vi "OpenFile_windows.vi"(0 "文件完整路径":path, 3 "文件父路径":path, 5 "文件全称":string) -> ()   [LabVIEW 2019]
panel:
  # "优先识别完整路径\n完整路径错误再识别拼接路径"
  # "用CMD来打开指定的文件，只要电脑的默认打开方式能打开对应的文件"
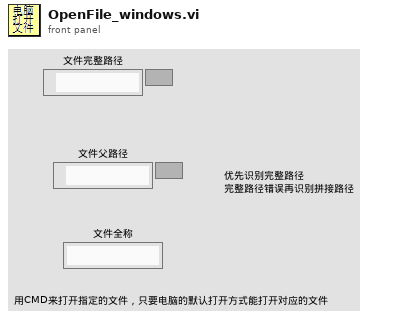
[diagram p1: front panel]
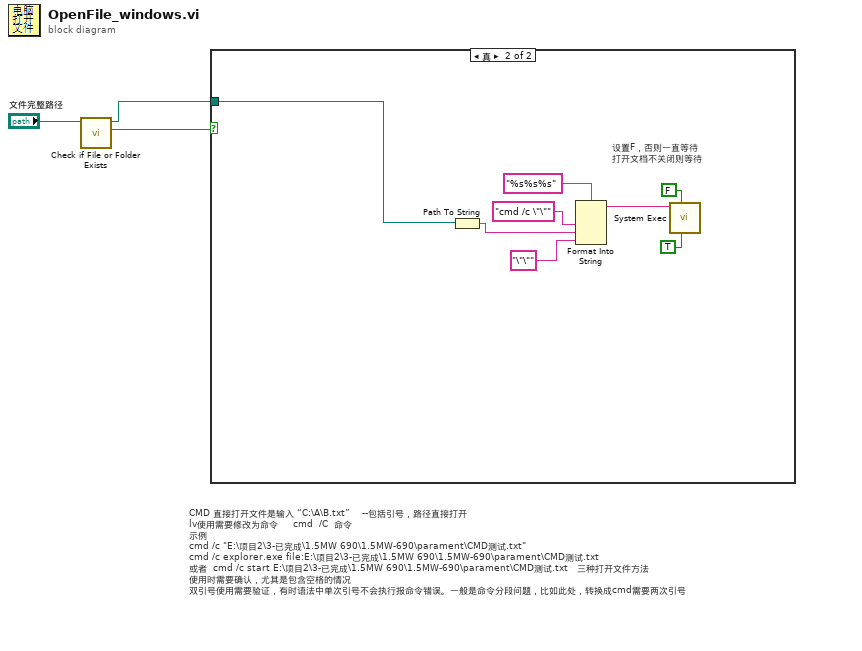
[diagram p0: block diagram]
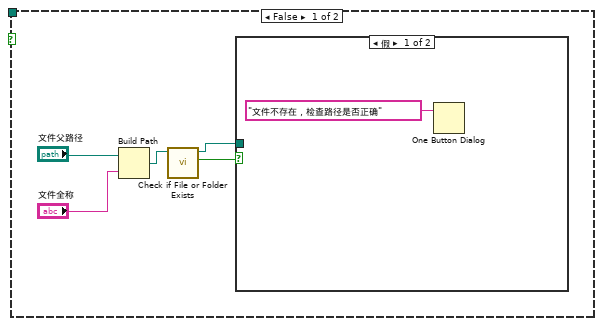
[diagram p2: hidden frame]
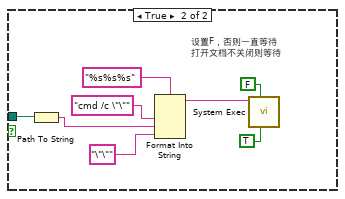
[diagram p3: hidden frame]
diagram:
  # "CMD 直接打开文件是输入 “C:\\A\\B.txt”    --包括引号，路径直接打开\nlv使用需要修改为命令     cmd  /C  命令\n示例\ncmd /c \"E:\\项目2\\3-已完成\\1.5MW 690\\1.5MW-690\\parament\\CMD测试.txt\" \ncmd /c explorer.exe file:E:\\项目2\\3-已完成\\1.5MW 690\\1.5MW-690\\parament\\CMD测试.txt         \n或者  cmd /c start E:\\项目2\\3-已完成\\1.5MW 690\\1.5MW-690\\parament\\CMD测试.txt   三种打开文件方法\n使用时需要确认，尤其是包含空格的情况\n双引号使用需要验证，有时语法中单次引号不会执行报命令错误。一般是命令分段问题，比如此处，转换成cmd需要两次引号"
  n1 = call <vilib>:"Check if File or Folder Exists.vi"("path"="文件完整路径") -> ("file or folder exists?"=w2:bool, "dup path"=w1:path)  [unwired: 8 in, 1 out]
  n2 = case shown="真" w2 {
    tunnel: w1 -> [_ w25]
    frame False {
      n3 = Build Path(base path="文件父路径", name or relative path="文件全称") -> (appended path=w6:path)
      n4 = call <vilib>:"Check if File or Folder Exists.vi"("path"=w6) -> ("file or folder exists?"=w5:bool, "dup path"=w4:path)  [unwired: 8 in, 1 out]
      n5 = case shown="假" w5 {
        tunnel: w4 -> [_ w15]
        frame False {
          n6 = One Button Dialog(message="文件不存在，检查路径是否正确" ("standard output")) -> ()  [unwired: 1 in, 1 out]
        }
        frame True {
          # "设置F，否则一直等待\n打开文档不关闭则等待"
          n7 = Path To String(path=w15) -> (string=w13:string)
          n8 = Format Into String(format string="%s%s%s" ("初始字符串"), "cmd /c \"\"" ("输入 1"), w13, "\"\"" ("输入 4")) -> (resulting string=w11:string)  [unwired: 2 in, 1 out]
          n9 = call <vilib>:"System Exec.vi"("run minimized? (F)"=TRUE, "wait until completion? (T)"=FALSE, "command line"=w11) -> ()  [unwired: 5 in, 4 out]
        }
      }
    }
    frame True {
      # "设置F，否则一直等待\n打开文档不关闭则等待"
      n10 = Path To String(path=w25) -> (string=w21:string)
      n11 = Format Into String(format string="%s%s%s" ("初始字符串"), "cmd /c \"\"" ("输入 1"), w21, "\"\"" ("输入 4")) -> (resulting string=w19:string)  [unwired: 2 in, 1 out]
      n12 = call <vilib>:"System Exec.vi"("run minimized? (F)"=TRUE, "wait until completion? (T)"=FALSE, "command line"=w19) -> ()  [unwired: 5 in, 4 out]
    }
  }
